vi "getInstanceConnStatus.vi"(8 "error in (no error)":errorcluster, 11 "tcpServer in":refnum<class "TcpServer.lvclass">) -> (0 "error out":errorcluster, 2 "ConnStatus":refnum<user-event>, 3 "tcpServer out":refnum<class "TcpServer.lvclass">)   [LabVIEW 2018, in "TcpServer.lvclass"]
doc: "Get the ConnStatus user event instance, to let Component know TcpServer is connected to all TCP clients."
uses:
  TcpServer.lvclass
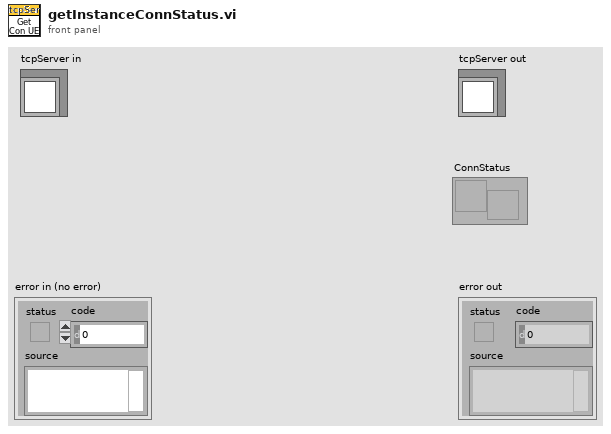
[diagram p1: front panel]
types:
  T1 = typedef "TcpServer.lvclass/userEventTypeDef.ctl" = cluster{"CmdRead":refnum<user-event>, "EvtRead":refnum<user-event>, "GenRead":refnum<user-event>, "ConnStatus":refnum<user-event>}
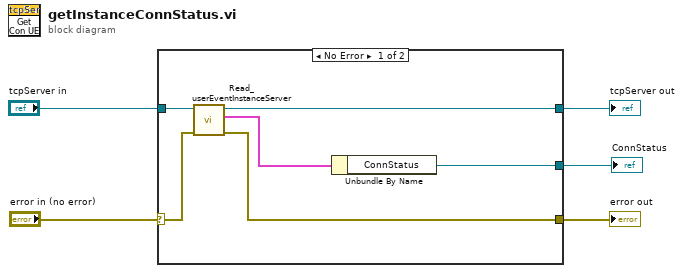
[diagram p0: block diagram]
diagram:
  n1 = case shown="No Error" "error in (no error)" {
    selector: "error in (no error)" -> [w9 w13]
    tunnel: [w7 w13] -> w4
    tunnel: [w10 w12] -> w2
    tunnel: "tcpServer in" -> [w11 w12]
    tunnel: [w6 _] -> w1
    frame No Error {
      n2 = call-dynamic "Read_userEventInstanceServer.vi"("error in (no error)"=w9, "TcpServer in"=w11) -> ("error out"=w7:errorcluster, "userEventInstanceServer"=w8:T1, "TcpServer out"=w10:refnum<class "TcpServer.lvclass">)  [unwired: 7 in]
      n3 = Unbundle By Name(w8) -> ("ConnStatus"=w6:refnum<user-event>)
    }
    frame Error {
    }
  }
  "error out" <- w4
  "tcpServer out" <- w2
  "ConnStatus" <- w1
